vi "testsuite arrays.vi"() -> ()   [LabVIEW 2018, in "LV-Julia_ZMQ-Roundtrip_lib.lvlib"]
uses:
  LV-Julia_ZMQ-Roundtrip_lib.lvlib
  05036e79-a137-49d8-b8bd-98c2707dfc19.vi
  42358c4e-b4d2-4416-9aa8-9e7cd75d6887.vi
panel:
  out "error out":errorcluster
  in  "dims0":u8=2 min=1 max=3
  in  "type0":i16
  out "out 1D":i16[](array[numeric])
  out "out 2D":i16[][](array[numeric])
  out "out 3D":i16[][][](array[numeric])
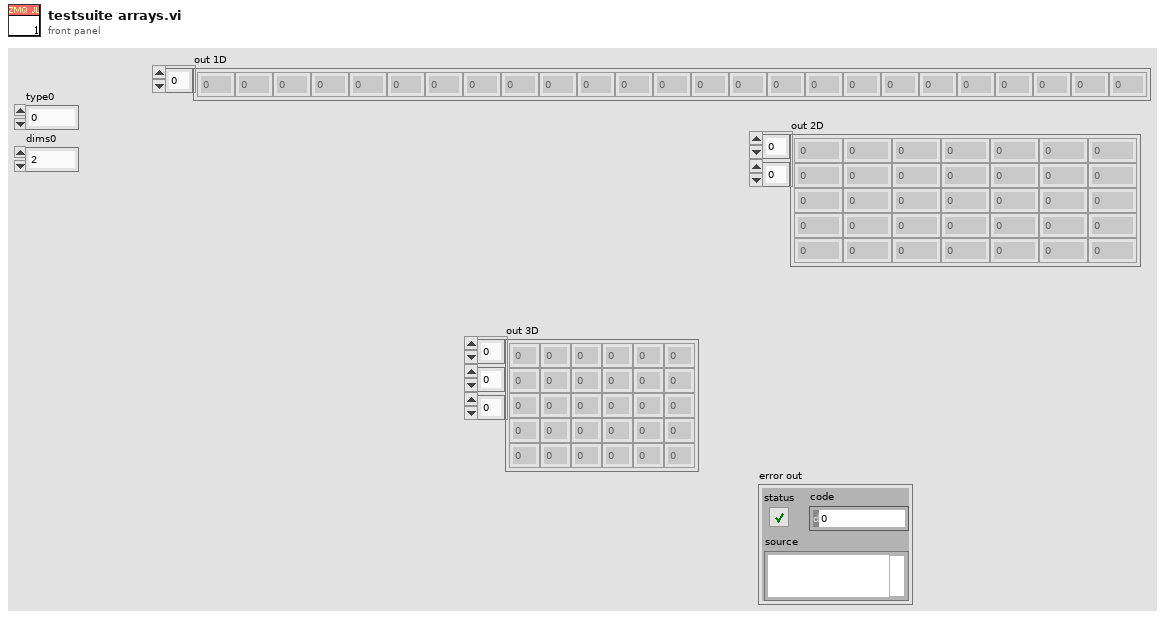
[diagram p1: front panel]
types:
  T1 = typedef "Bindata&description.ctl" = cluster{"bindata_descr":T2[], "bindata":u8[]}
  T2 = typedef "LV-Julia_ZMQ-Roundtrip_lib.lvlib/Bindata description.ctl" = cluster{"nofbytes":i32, "numtype":string, "start":i32, "arrdims":i32[], "kwarg_name":string, "category":string}
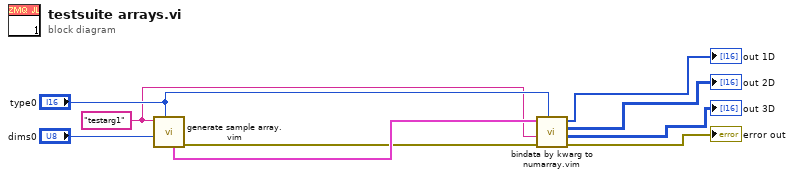
[diagram p0: block diagram]
diagram:
  w1 = "testarg1" ("kwarg_name")
  n1 = call "generate sample array.vim"("type"="type0", "dims"="dims0", "kwarg_name"=w1) -> ("error out"=w8:errorcluster, "Bindata & descr out"=w9:T1)  [unwired: 3 in, 4 out]
  n2 = call "bindata by kwarg to numarray.vim"("type in"="type0", "error in (no error)"=w8, "kwarg_name"=w1, "Bindata & descr in"=w9) -> ("error out"=→"error out":errorcluster, "numarray 3D"=→"out 3D":i16[][][], "numarray 2D"=→"out 2D":i16[][], "numarray 1D"=→"out 1D":i16[])  [unwired: 4 in]
